vi "Untitled 3 (SubVI).vi"(6 "RawCO2s":dbl[](array[numeric]), 10 "Daq Needed":T1 {"Current Settings"."Pump" items=["Pump 0", "Pump 1", "Pump 2", "Pump 3", "Pump 4", "Pump 5"]; "Current Settings"."Chart X axis Timescale" min=20 max=180 step=1; "Current Settings"."RunTime Mode Settings"."Exp. Gas Tank" items=["0.07", "0.031", "0.877", "1.863", "3.881", "5.790", "7.688", "6.000"]; "Current Settings"."RunTime Mode Settings"."Insp. Gas Tank" items=["0.07", "0.031", "0.877", "1.863", "3.881", "5.790", "7.688", "6.000"]; "Current Settings"."RunTime Mode Settings"."I:E Ratio" max=30 scale=0.0..7.0; "Current Settings"."RunTime Mode Settings"."Resp Rate Brpm" min=0 max=30 format="%.2f"; "Current Settings"."TE#2 Configuration"."Serial Port"."XOFF Char" format="%.0x"; "Current Settings"."TE#2 Configuration"."Serial Port"."XON Char" format="%.0x"; "Current Settings"."TE#2 Configuration"."Serial Port"."flow control" items=["None"=0, "XON/XOFF"=1, "RTS/CTS"=2, "DTR/DSR"=4]; "Current Settings"."TE#2 Configuration"."Serial Port"."stop bits" items=["1.0"=10, "1.5"=15, "2.0"=20]; "Current Settings"."TE#2 Configuration"."Serial Port"."data bits" min=5 max=8 step=1; "Current Settings"."TE#2 Configuration"."Serial Port"."baud rate" items=["75"=75, "110"=110, "134"=134, "150"=150, "300"=300, "600"=600, "1200"=1200, "1800"=1800, "2400"=2400, "4800"=4800, "7200"=7200, "9600"=9600, "14400"=14400, "19200"=19200, "28800"=28800, "38400"=38400, "56000"=56000, "57600"=57600, "115200"=115200, "128000"=128000, "230400"=230400]; "Current Settings"."TE#2 Configuration"."Serial Port"."termination char" format="%.0x"; "Current Settings"."TE#1 Configuration"."Serial Port"."XOFF Char" format="%.0x"; "Current Settings"."TE#1 Configuration"."Serial Port"."XON Char" format="%.0x"; "Current Settings"."TE#1 Configuration"."Serial Port"."flow control" items=["None"=0, "XON/XOFF"=1, "RTS/CTS"=2, "DTR/DSR"=4]; "Current Settings"."TE#1 Configuration"."Serial Port"."stop bits" items=["1.0"=10, "1.5"=15, "2.0"=20]; "Current Settings"."TE#1 Configuration"."Serial Port"."data bits" min=5 max=8 step=1; "Current Settings"."TE#1 Configuration"."Serial Port"."baud rate" items=["75"=75, "110"=110, "134"=134, "150"=150, "300"=300, "600"=600, "1200"=1200, "1800"=1800, "2400"=2400, "4800"=4800, "7200"=7200, "9600"=9600, "14400"=14400, "19200"=19200, "28800"=28800, "38400"=38400, "56000"=56000, "57600"=57600, "115200"=115200, "128000"=128000, "230400"=230400]; "Current Settings"."TE#1 Configuration"."Serial Port"."termination char" format="%.0x"; "Current Settings"."Capnometer Configuration"."Device" items=["None", "TidalWave", "LoFlow / Canary", "Capnogard"]; "Current Settings"."Capnometer Configuration"."Serial Port"."XOFF Char" format="%.0x"; "Current Settings"."Capnometer Configuration"."Serial Port"."XON Char" format="%.0x"; "Current Settings"."Capnometer Configuration"."Serial Port"."flow control" items=["None"=0, "XON/XOFF"=1, "RTS/CTS"=2, "DTR/DSR"=4]; "Current Settings"."Capnometer Configuration"."Serial Port"."stop bits" items=["1.0"=10, "1.5"=15, "2.0"=20]; "Current Settings"."Capnometer Configuration"."Serial Port"."data bits" min=5 max=8 step=1; "Current Settings"."Capnometer Configuration"."Serial Port"."baud rate" items=["75"=75, "110"=110, "134"=134, "150"=150, "300"=300, "600"=600, "1200"=1200, "1800"=1800, "2400"=2400, "4800"=4800, "7200"=7200, "9600"=9600, "14400"=14400, "19200"=19200, "28800"=28800, "38400"=38400, "56000"=56000, "57600"=57600, "115200"=115200, "128000"=128000, "230400"=230400]; "Current Settings"."Capnometer Configuration"."Serial Port"."termination char" format="%.0x"; "Current Settings"."DAQx Settings"."Analog Output Settings (Volts)" format="%#.3g"; "Current Settings"."DAQx Settings"."Duty Cycle" min=10.0 max=90.0 format="%.1g"; "Current Settings"."DAQx Settings"."Frequency" min=20.0 max=200.0; "Current Settings"."DataLogging Settings"."Data File Duration (Minutes)" min=2 max=200 format="%#.2g"; "Current Settings"."Calibration Settings"."Tolerance #2" min=2 max=4096; "Current Settings"."Calibration Settings"."Cal. Average" min=2 max=4096; "Current Settings"."Test Settings"."Test Sensor ID" items=["(select)", "RB", "YC", "", "Other"]}, 11 "Use Channel":u8) -> (2 "Array":dbl[][](array[numeric]), 3 "Raw CO2":dbl)   [LabVIEW 2015]
uses:
  Controls/DAQ Needed.ctl
  Controls/Processed Variables.ctl
  Controls/AirPump Controls.ctl
  Controls/IE Ratio knob.ctl
  Controls/UI Settings.ctl
  Controls/Aux CO2 Control.ctl
  Controls/Serial Visa Control.ctl
  Controls/Aux CO2 Selector.ctl
  Controls/Aux TE Control.ctl
  Controls/Queues And Others.ctl
panel:
  # "Note: Setting Brpm to zero will\ndisable Insp / Exp digital output."
  # "mmHg"
  # "pts"
  # "tolerance"
  # "AN5 (Temp 1)"
  # "AN6 (Temp 2)"
  # "AN7 (Temp 3)"
  # "AN8 (T FET)"
  # "AN0 (T POT)"
  # "Tref (Set Pt))"
  # "(Spare)"
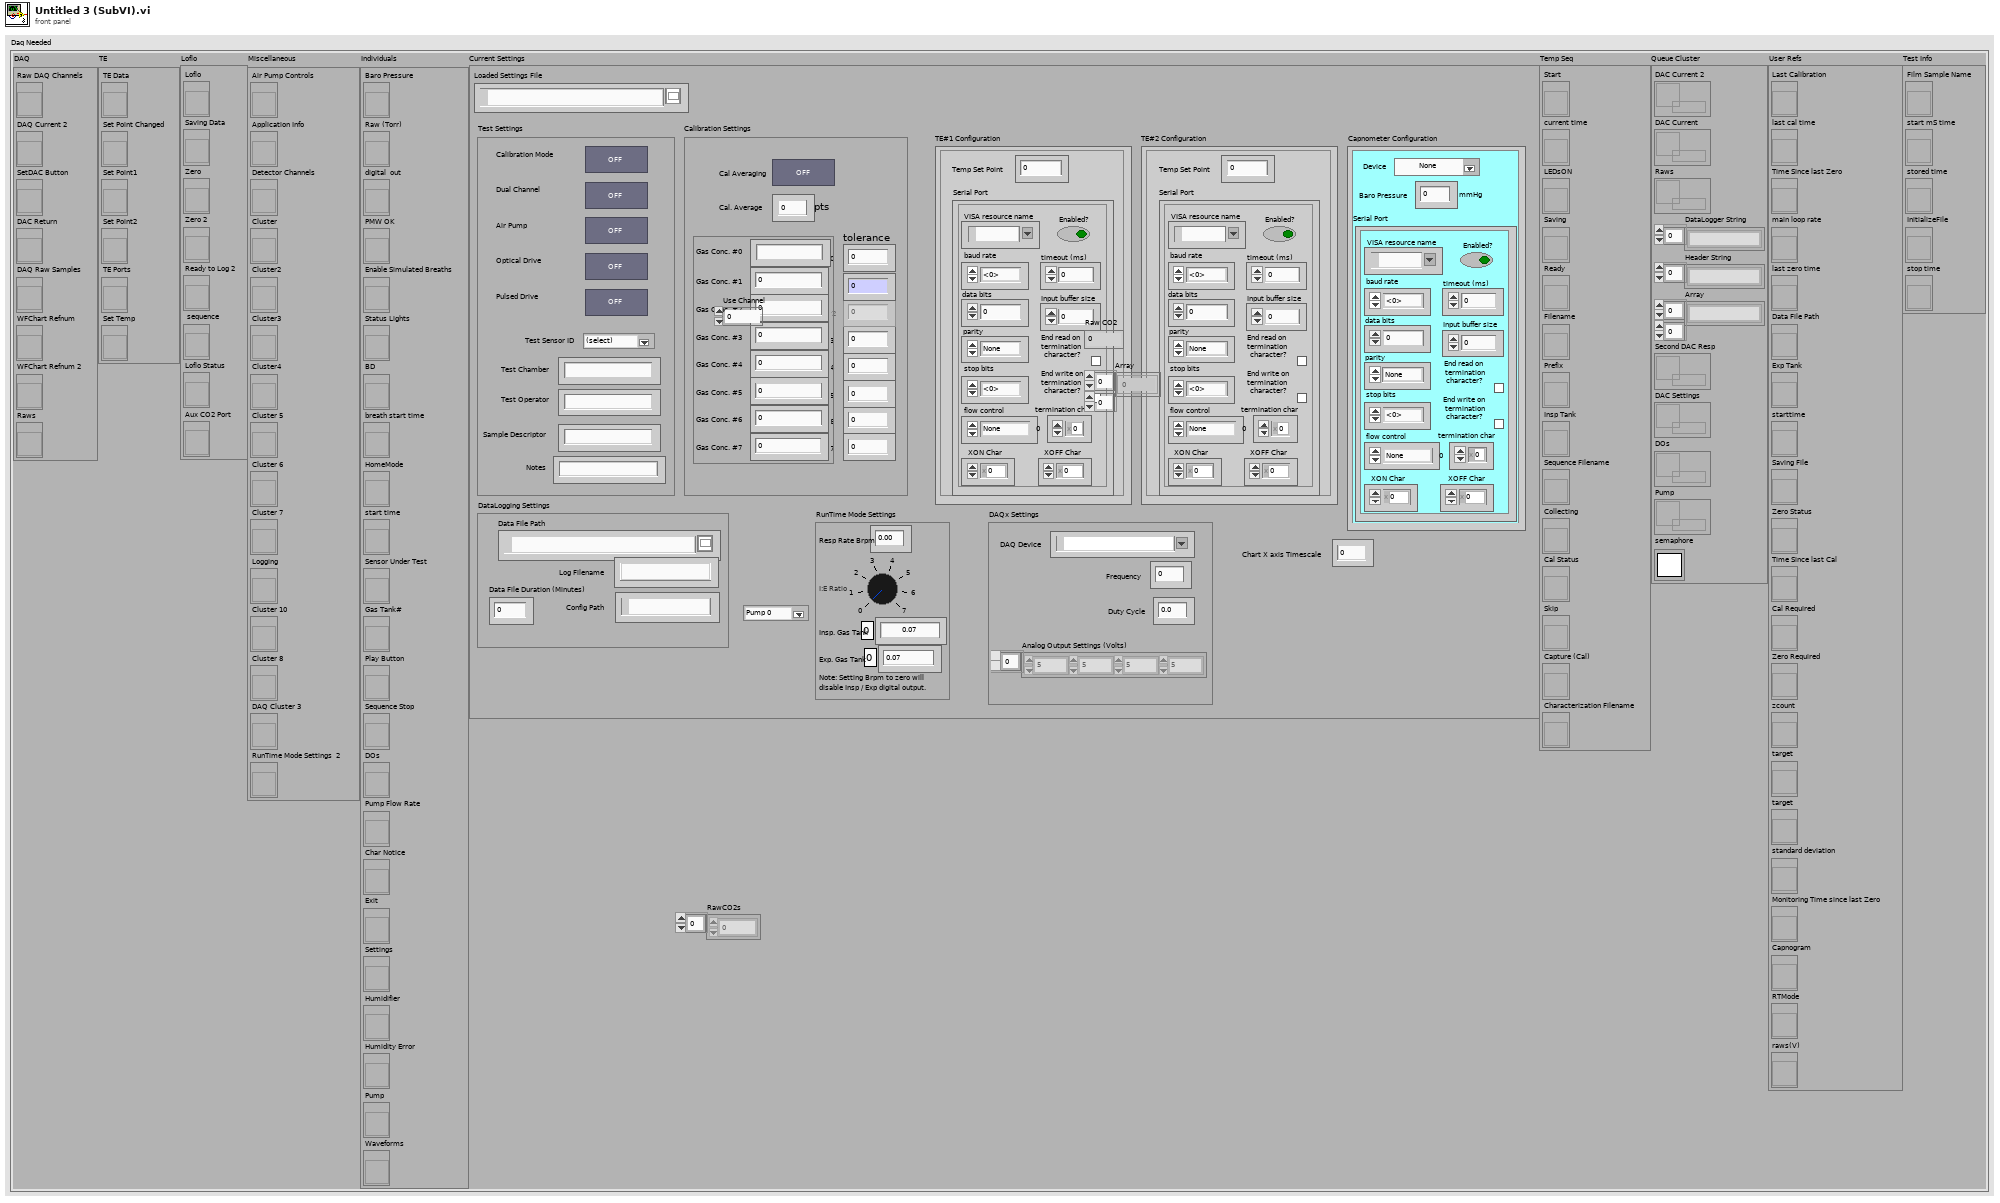
[diagram p1: front panel]
types:
  T1 = typedef "DAQ Needed.ctl" = cluster{"DAQ":cluster{"Raw DAQ Channels":refnum<vi>, "DAQ Current 2":refnum<vi>, "SetDAC Button":refnum<vi>, "DAC Return":refnum<vi>, "DAQ Raw Samples":refnum<vi>, "WFChart Refnum":refnum<vi>, "WFChart Refnum 2":refnum<vi>, "Raws":refnum<vi>}, "TE":cluster{"TE Data":refnum<vi>, "Set Point Changed":refnum<vi>, "Set Point1":refnum<vi>, "Set Point2":refnum<vi>, "TE Ports":refnum<vi>, "Set Temp":refnum<vi>}, "Loflo":cluster{"Loflo":refnum<vi>, "Saving Data":refnum<vi>, "Zero":refnum<vi>, "Zero 2":refnum<vi>, "Ready to Log 2":refnum<vi>, " sequence":refnum<vi>, "Loflo Status ":refnum<vi>, "Aux CO2 Port":refnum<vi>}, "Miscellaneous":cluster{"Air Pump Controls":refnum<vi>, "Application Info":refnum<vi>, "Detector Channels ":refnum<vi>, "Cluster":refnum<vi>, "Cluster2":refnum<vi>, "Cluster3":refnum<vi>, "Cluster4":refnum<vi>, "Cluster 5":refnum<vi>, "Cluster 6":refnum<vi>, "Cluster 7":refnum<vi>, "Logging":refnum<vi>, "Cluster 10":refnum<vi>, "Cluster 8":refnum<vi>, "DAQ Cluster 3":refnum<vi>, "RunTime Mode Settings  2":refnum<vi>}, "Individuals":cluster{"Baro Pressure":refnum<vi>, "Raw (Torr)":refnum<vi>, "digital  out":refnum<vi>, "PMW OK":refnum<vi>, "Enable Simulated Breaths":refnum<vi>, "Status Lights":refnum<vi>, "BD":refnum<vi>, "breath start time":refnum<vi>, "HomeMode":refnum<vi>, "start time":refnum<vi>, "Sensor Under Test":refnum<vi>, "Gas Tank#":refnum<vi>, "Play Button":refnum<vi>, "Sequence Stop":refnum<vi>, "DOs":refnum<vi>, "Pump Flow Rate":refnum<vi>, "Char Notice":refnum<vi>, "Exit":refnum<vi>, "Settings":refnum<vi>, "Humidifier":refnum<vi>, "Humidity Error":refnum<vi>, "Pump":refnum<vi>, "Waveforms":refnum<vi>}, "Current Settings":T2, "Temp Seq":cluster{"Start":refnum<vi>, "current time":refnum<vi>, "LEDsON":refnum<vi>, "Saving":refnum<vi>, "Ready":refnum<vi>, "Filename":refnum<vi>, "Prefix":refnum<vi>, "Insp Tank":refnum<vi>, "Sequence Filename":refnum<vi>, "Collecting":refnum<vi>, "Cal Status":refnum<vi>, "Skip":refnum<vi>, "Capture (Cal)":refnum<vi>, "Characterization Filename":refnum<vi>}, "Queue Cluster":T7, "User Refs":cluster{"Last Calibration":refnum<vi>, "last cal time":refnum<vi>, "Time Since last Zero":refnum<vi>, "main loop rate":refnum<vi>, "last zero time":refnum<vi>, "Data File Path":refnum<vi>, "Exp Tank":refnum<vi>, "starttime":refnum<vi>, "Saving File":refnum<vi>, "Zero Status":refnum<vi>, "Time Since last Cal":refnum<vi>, "Cal Required":refnum<vi>, "Zero Required":refnum<vi>, "zcount":refnum<vi>, "target":refnum<vi>, "target":refnum<vi>, "standard deviation":refnum<vi>, "Monitoring Time since last Zero":refnum<vi>, "Capnogram":refnum<vi>, "RTMode":refnum<vi>, "raws(V)":refnum<vi>}, "Test Info":cluster{"Film Sample Name":refnum<vi>, "start mS time":refnum<vi>, "stored time":refnum<vi>, "InitializeFile":refnum<vi>, "stop time":refnum<vi>}}
  T2 = typedef "UI Settings.ctl" = cluster{"Loaded Settings File":path, "Test Settings":cluster{"Dual Channel":bool, "Air Pump":bool, "Optical Drive":bool, "Pulsed Drive":bool, "Calibration Mode":bool, "Test Sensor ID":u16, "Test Chamber":string, "Test Operator":string, "Sample Descriptor":string, "Notes":string}, "Calibration Settings":cluster{"Cal. Average":u16, "Cal Averaging":bool, "Tolerance #0":sgl, "Tolerance #7":sgl, "Tolerance #6":sgl, "Tolerance #5":sgl, "Tolerance #4":sgl, "Tolerance #3":sgl, "Tolerance #2":sgl, "Tolerance #1":sgl, "Gas Tank Settings":cluster{"Gas Conc. #0":string, "Gas Conc. #1":sgl, "Gas Conc. #2":sgl, "Gas Conc. #3":sgl, "Gas Conc. #4":sgl, "Gas Conc. #5":sgl, "Gas Conc. #6":sgl, "Gas Conc. #7":sgl}}, "DataLogging Settings":cluster{"Data File Path":path, "Data File Duration (Minutes)":sgl, "Log Filename":string, "Config Path":path}, "DAQx Settings":cluster{"DAQ Device":tag, "Frequency":dbl, "Duty Cycle":dbl, "Analog Output Settings (Volts)":sgl[]}, "Capnometer Configuration":T3, "TE#1 Configuration":T6, "TE#2 Configuration":T6, "RunTime Mode Settings ":cluster{"Resp Rate Brpm ":sgl, "I:E Ratio":u8, "Insp. Gas Tank":u16, "Exp. Gas Tank":u16}, "Chart X axis Timescale":u16, "Pump":u16}
  T3 = typedef "Aux CO2 Control.ctl" = cluster{"Serial Port":T4, "Baro Pressure":u32, "Device":T5}
  T4 = typedef "Serial Visa Control.ctl" = cluster{"termination char":u8, "End read on termination character?":bool, "Enabled?":bool, "VISA resource name":refnum<visa-resource-name>, "baud rate":u32, "data bits":u16, "parity":enum16{"None", "Odd", "Even", "Mark", "Space"}, "stop bits":u16, "flow control":u16, "timeout (ms)":u32, "Input buffer size":u32, "End write on termination character?":bool, "XON Char":u8, "XOFF Char":u8}
  T5 = typedef "Aux CO2 Selector.ctl" = u16
  T6 = typedef "Aux TE Control.ctl" = cluster{"Temp Set Point":sgl, "Serial Port":T4}
  T7 = typedef "Queues And Others.ctl" = cluster{"DAC Current 2":refnum<queue>, "DAC Current":refnum<queue>, "Raws":refnum<queue>, "DataLogger String":string[], "Header String":string[], "Array":string[][], "Second DAC Resp":refnum<queue>, "DAC Settings":refnum<queue>, "DOs":refnum<queue>, "Pump":refnum<queue>, "semaphore":T8}
  T8 = typedef "Semaphore RefNum" = refnum<k1>
  T9 = typedef "IE Ratio knob.ctl" = u8
  T10 = cluster{"pk":sgl, "RawCO2":sgl, "Uncal'd":sgl, "Avg_Hum":sgl, "Avg'd CO2":sgl, "Home_CO2":sgl, "Home_Ref":sgl, "Home_Hum":sgl, " Home Temp":dbl, "Pump Flow Rate":u16, "I:E Ratio":T9, "Brpm":sgl, "Sim Breaths":bool, "GasTank":u8}
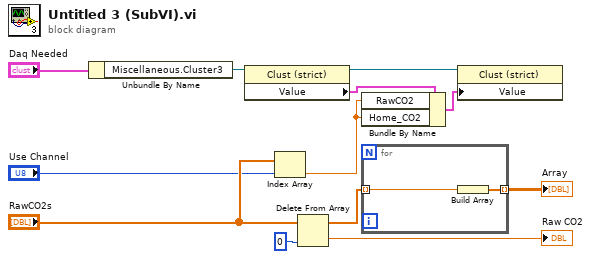
[diagram p0: block diagram]
diagram:
  n1 = Unbundle By Name("Daq Needed") -> ("Miscellaneous.Cluster3"=w8:refnum<vi>)
  n2 = property class="Clust (strict)"(reference=w8) -> (reference out=w9:refnum<vi>, "Value"=w10:T10)  [unwired: 1 in, 1 out]
  n3 = Index Array(array="RawCO2s", index="Use Channel") -> (element=w12:dbl)
  n4 = Delete From Array(array="RawCO2s", index=0) -> (deleted portion=→"Raw CO2":dbl, array with subset deleted=w4:dbl[])  [unwired: 1 in]
  n5 = Bundle By Name(cluster=w10, "RawCO2"=w12, "Home_CO2"=w12) -> (w11:T10)
  n6 = for {
    tunnel: w4 -> [w14] mode=indexing
    tunnel: [w13] -> w2 mode=indexing
    n7 = Build Array(w14) -> (w13:dbl[])
  }
  "Array" <- w2
  n8 = property class="Clust (strict)"(reference=w9, "Value"=w11) -> ()  [unwired: 1 in, 2 out]
